vi "ActionVIOnLoad.vi"(8 "error in (no error)":errorcluster, 11 "Device Item Ref in":T1 format="%.0x") -> (0 "error out":errorcluster, 3 "Device Item Ref out":T1 format="%.0x")   [LabVIEW 2020, in "SLSC EDS System Explorer.lvlib"]
uses:
  SLSC EDS System Explorer.lvlib
  <vilib>/NI VeriStand/Custom Device API/Custom Device Item Ref.ctl
  NationalInstruments.VeriStand.SystemDefinitionAPI
  Shared/Constants.vi
  <vilib>/NI VeriStand/Custom Device API/Custom Device API.lvlib
  Shared/SLSC EDS Shared.lvlib
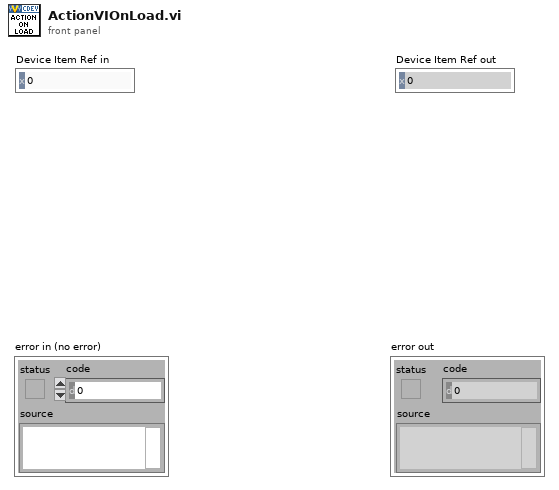
[diagram p1: front panel]
types:
  T1 = typedef "Custom Device API.lvlib/Custom Device Item Ref.ctl" = u64
  T2 = typedef "Custom Device API.lvlib/Custom Device Item Info.ctl" = cluster{"Name":string, "Is Channel":bool, "GUID":string, "Is Waveform":bool}
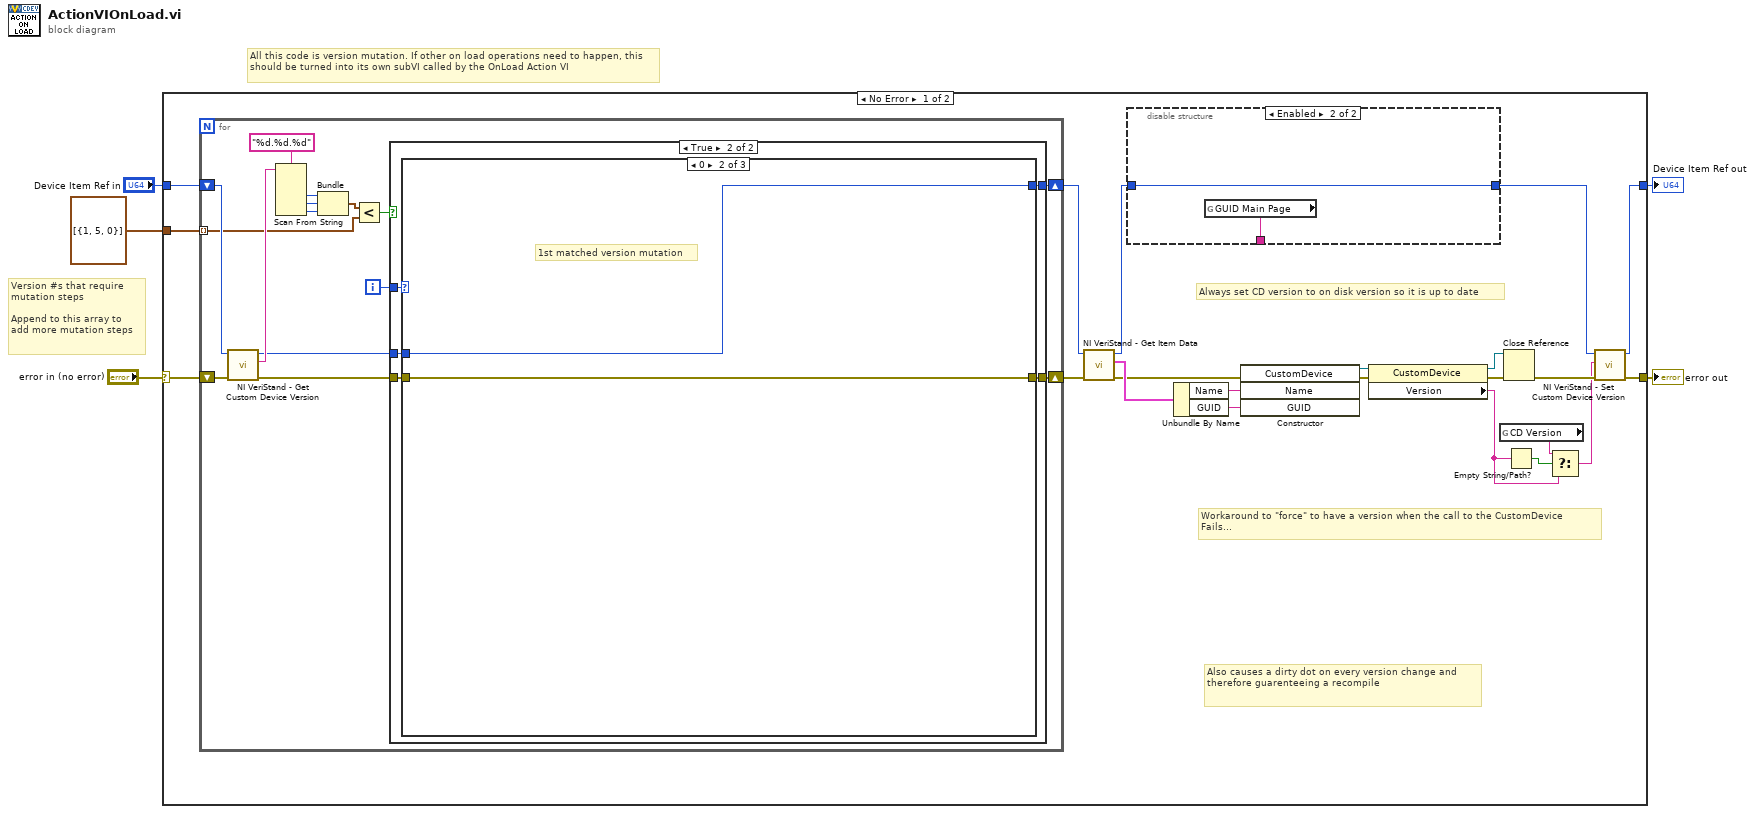
[diagram p0: block diagram]
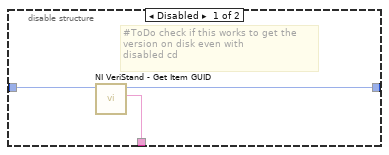
[diagram p2: hidden frame]
diagram:
  # "All this code is version mutation. If other on load operations need to happen, this should be turned into its own subVI called by the OnLoad Action VI"
  # "Version #s that require\nmutation steps\n\nAppend to this array to\nadd more mutation steps"
  n1 = case shown="No Error" "error in (no error)" {
    selector: "error in (no error)" -> [w26 w62]
    tunnel: [w19 w62] -> w4
    tunnel: "Device Item Ref in" -> [w25 w61]
    tunnel: [w18 w61] -> w2
    tunnel: cluster{i32, i32, i32}[] [{1, 5, 0}] -> [w27 _]
    frame No Error {
      # "Workaround to \"force\" to have a version when the call to the CustomDevice\nFails..."
      # "Also causes a dirty dot on every version change and therefore guarenteeing a recompile"
      # "Always set CD version to on disk version so it is up to date"
      n2 = for {
        tunnel: w27 -> [w34] mode=indexing
        shift-right: [w38] -> w16
        shift-left: w26 -> [w43]
        shift-right: [w36] -> w15
        shift-left: w25 -> [w42]
        i -> [w35]
        n3 = call <vilib>:"NI VeriStand - Get Custom Device Version.vi"("error in (no error)"=w43, "Device Ref in"=w42) -> ("error out"=w39:errorcluster, "Value"=w41:string, "Device Ref out"=w37:T1)  [unwired: 7 in]
        n4 = Scan From String(format string="%d.%d.%d", input string=w41) -> (output 1=w45:i32, output 2=w46:i32, output 3=w33:i32)  [unwired: 5 in, 3 out]
        n5 = Bundle(w45, w46, w33) -> (w47:cluster{i32, i32, i32})  [unwired: 1 in]
        n6 = Less?(x=w47, y=w34) -> (x < y?=w40:bool)
        n7 = case shown="True" w40 {
          tunnel: w39 -> [w49 w54]
          tunnel: [w49 w53] -> w38
          tunnel: w37 -> [w48 w50]
          tunnel: [w48 w51] -> w36
          tunnel: w35 -> [_ w52]
          frame False {
          }
          frame True {
            n8 = case shown="0" w52 {
              tunnel: w54 -> [w56 w57 w59]
              tunnel: [w56 w57 w59] -> w53
              tunnel: [w55 w58 w60] -> w51
              tunnel: w50 -> [w55 w58 w60]
              frame Default {
              }
              frame 0 {
                # "1st matched version mutation"
              }
              frame 1 {
                # "2nd matched version mutation"
              }
            }
          }
        }
      }
      n9 = call <vilib>:"NI VeriStand - Get Item Data.vi"("error in (no error)"=w16, "Item Ref in"=w15) -> ("error out"=w13:errorcluster, "Item Info"=w17:T2, "Item Ref out"=w14:T1)  [unwired: 6 in, 1 out]
      n10 = disable-structure shown="Enabled" {
        disable-tunnel: w14 -> [w30 w32]
        disable-tunnel: [w29 w31] -> _
        disable-tunnel: [w28 w32] -> w10
        frame Disabled {
          # "#ToDo check if this works to get the \nversion on disk even with \ndisabled cd"
          n11 = call <vilib>:"NI VeriStand - Get Item GUID.vi"("Item Ref in"=w30) -> ("GUID"=w29:string, "Item Ref out"=w28:T1)  [unwired: 8 in, 1 out]
        }
        frame Enabled {
          n12 = global read "Constants.vi" "GUID Main Page"() -> (w31:string)
        }
      }
      n13 = Unbundle By Name(w17) -> ("Name"=w12:string, "GUID"=w11:string)
      n14 = constructor class="CustomDevice"(error in=w13, "Name"=w12, "GUID"=w11) -> (reference out=w24:refnum<k24>, error out=w23:errorcluster)  [unwired: 2 in, 3 out]
      n15 = property class="CustomDevice"(reference=w24, error in=w23) -> (reference out=w21:refnum<k24>, error out=w22:errorcluster, "Version"=w7:string)
      n16 = global read "Constants.vi" "CD Version"() -> (w8:string)
      n17 = Close Reference(reference=w21, error in (no error)=w22) -> (error out=w20:errorcluster)
      n18 = Empty String/Path?(string/path=w7) -> (empty?=w9:bool)
      n19 = Select(t=w8, s=w9, f=w7) -> (s? t:f=w6:string)
      n20 = call <vilib>:"NI VeriStand - Set Custom Device Version.vi"("error in (no error)"=w20, "Value"=w6, "Device Ref in"=w10) -> ("error out"=w19:errorcluster, "Device Ref out"=w18:T1)  [unwired: 7 in]
    }
    frame Error {
    }
  }
  "error out" <- w4
  "Device Item Ref out" <- w2
